vi "AM_Freq_Resp_Sweep.vi"(4 "error in":errorcluster, 5 "fdelta / kHz":dbl, 6 "flow / kHz":dbl, 7 "fhigh / kHz":dbl, 8 "VISA resource name 2":refnum<visa-resource-name>) -> (0 "error out":errorcluster, 1 "Rdata":dbl[](array[numeric]), 2 "Fdata":dbl[](array[numeric]), 3 "VISA resource name 3":refnum<visa-resource-name>)   [LabVIEW 2019]
doc: "Perform frequency response measurement using Arduino Micro + Spark Fun MiniGen\n\nR. Sheehan 18 - 11 - 2020"
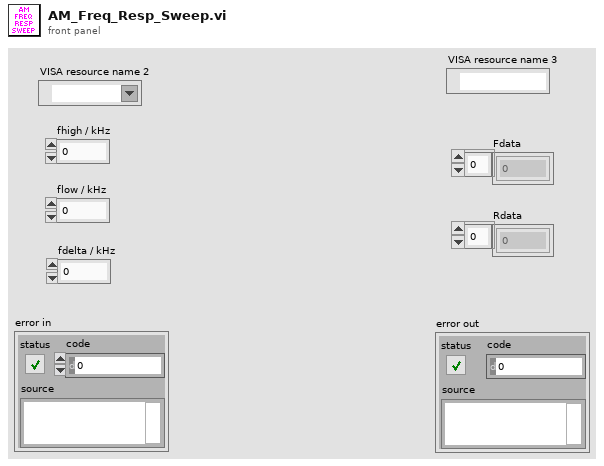
[diagram p1: front panel]
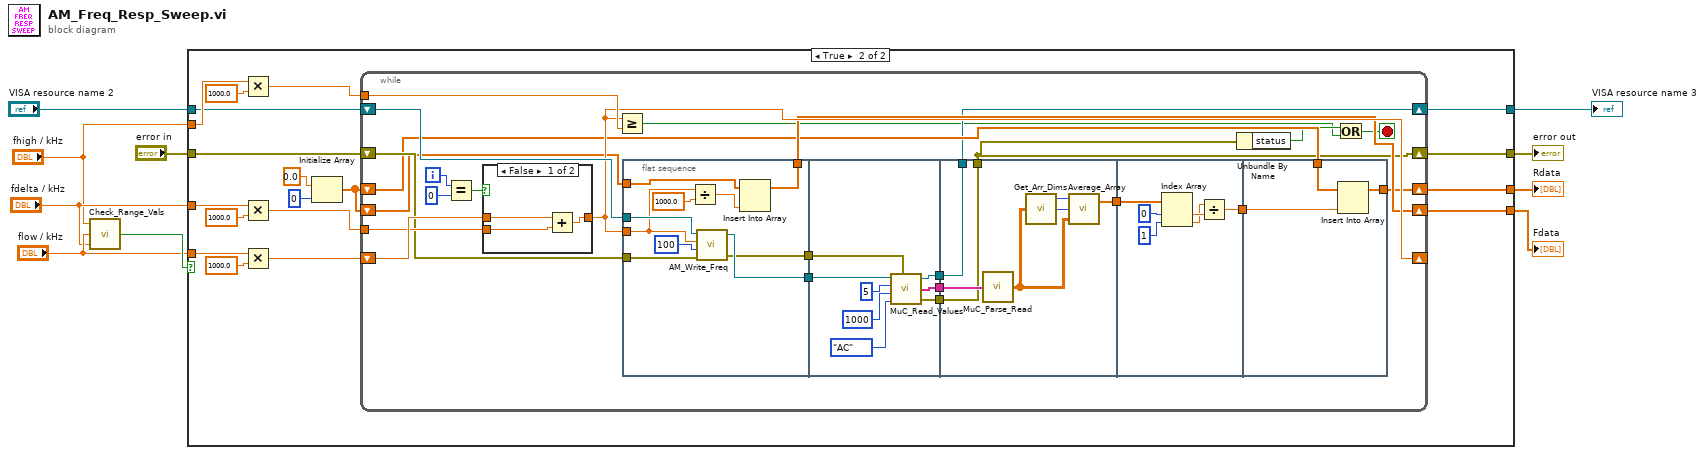
[diagram p0: block diagram]
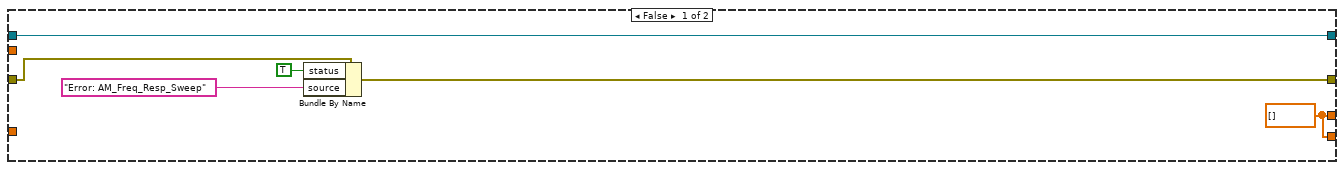
[diagram p2: hidden frame]
diagram:
  n1 = call "Check_Range_Vals.vi"("Increment"="fdelta / kHz", "Lower Limit"="flow / kHz", "Upper Limit"="fhigh / kHz") -> ("Bounds Are Good"=w10:bool)
  n2 = case shown="True" w10 {
    tunnel: "flow / kHz" -> [_ w30]
    tunnel: "fdelta / kHz" -> [_ w27]
    tunnel: "fhigh / kHz" -> [_ w34]
    tunnel: "VISA resource name 2" -> [w16 w25]
    tunnel: "error in" -> [w14 w24]
    tunnel: [w16 w18] -> w4
    tunnel: [w13 w17] -> w3
    tunnel: [w15 w20] -> w2
    tunnel: [w15 w19] -> w1
    frame False {
      w15 = dbl[] []
      n3 = Bundle By Name(cluster=w14, "status"=TRUE, "source"="Error: AM_Freq_Resp_Sweep") -> (w13:errorcluster)
    }
    frame True {
      n4 = Multiply(x=w34, y=1000.0) -> (x*y=w32:dbl)
      n5 = Multiply(x=w27, y=1000.0) -> (x*y=w26:dbl)
      n6 = Multiply(x=w30, y=1000.0) -> (x*y=w29:dbl)
      n7 = Initialize Array(0.0 ("element"), 0 ("dimension size")) -> (w21:dbl[])
      n8 = while {
        shift-right: [w45] -> _
        shift-left: w29 -> [w56]
        tunnel: w26 -> [w55]
        tunnel: w32 -> [w54]
        shift-right: [w41] -> w19
        shift-left: w21 -> [w42]
        shift-right: [w43] -> w20
        shift-left: w21 -> [w44]
        shift-right: [w39] -> w18
        shift-left: w25 -> [w47]
        shift-right: [w38] -> w17
        shift-left: w24 -> [w46]
        i -> [w58]
        stop <- w35 stop-if-true
        n9 = Equal?(x=w58, y=0) -> (x = y?=w59:bool)
        n10 = case shown="False" w59 {
          tunnel: w56 -> [w96 w97]
          tunnel: [w94 w97] -> w45
          tunnel: w55 -> [w95 _]
          frame False {
            n11 = Add(x=w96, y=w95) -> (x+y=w94:dbl)
          }
          frame True {
          }
        }
        n12 = Greater Or Equal?(x=w45, y=w54) -> (x >= y?=w36:bool)
        n13 = flat-sequence {
          tunnel: [w69] -> w53
          tunnel: [w68] -> w52
          tunnel: w47 -> [w67]
          tunnel: w46 -> [w66]
          tunnel: w45 -> [w62]
          tunnel: w44 -> [w65]
          tunnel: [w64] -> w43
          tunnel: w53 -> [w75]
          tunnel: [w77] -> w51
          tunnel: w52 -> [w76]
          tunnel: [w74] -> w50
          tunnel: [w73] -> w49
          tunnel: w51 -> [w84]
          tunnel: w50 -> [w79]
          tunnel: [w80] -> w48
          tunnel: w49 -> [w78]
          tunnel: [w79] -> w39
          tunnel: [w78] -> w38
          tunnel: w48 -> [w90]
          tunnel: [w85] -> w40
          tunnel: w42 -> [w93]
          tunnel: [w92] -> w41
          tunnel: w40 -> [w91]
          frame #0 {
            n14 = Divide(x=w62, y=1000.0) -> (x/y=w60:dbl)
            n15 = call "AM_Write_Freq.vi"("error in (no error)"=w66, "Delay / ms"=u32 100, "f / Hz"=w62, "VISA resource name"=w67) -> ("error out"=w68:errorcluster, "VISA resource name 2"=w69:refnum<visa-resource-name>)  [unwired: 1 out]
            n16 = Insert Into Array(array=w65, new element=w60) -> (w64:dbl[])  [unwired: 1 in]
          }
          frame #1 {
            n17 = call "MuC_Read_Values.vi"("VISA resource name"=w75, "Nreads"=5, "Delay (ms)"=u32 1000, "Read Type"=enum16{"DC", "AC"}."AC", "error in (no error)"=w76) -> ("VISA resource name 2"=w74:refnum<visa-resource-name>, "Buffer Data"=w77:string[], "error out"=w73:errorcluster)
          }
          frame #2 {
            n18 = call "MuC_Parse_Read.vi"("Buffer Data"=w84) -> ("Data"=w83:dbl[][])
            n19 = call "Get_Arr_Dims.vi"("Data"=w83) -> ("N Rows"=w82:i32, "N Cols"=w81:i32)  [unwired: 1 out]
            n20 = call "Average_Array.vi"("Array"=w83, "Ncolumns"=w81, "Nrows"=w82) -> ("Average"=w80:dbl[])  [unwired: 1 out]
          }
          frame #3 {
            n21 = Index Array(array=w90, index #1=0 ("index"), index #2=1 ("index")) -> (element #1=w87:dbl, element #2=w86:dbl)
            n22 = Divide(x=w86, y=w87) -> (x/y=w85:dbl)
          }
          frame #4 {
            n23 = Insert Into Array(array=w93, new element=w91) -> (w92:dbl[])  [unwired: 1 in]
          }
        }
        n24 = Unbundle By Name(w38) -> ("status"=w37:bool)
        n25 = Or(x=w37, y=w36) -> (x .or. y?=w35:bool)
      }
    }
  }
  "VISA resource name 3" <- w4
  "error out" <- w3
  "Fdata" <- w2
  "Rdata" <- w1
